vi "Create Reference.vi"(8 "Error In":errorcluster, 11 "Reader In":refnum<class "Reader.lvclass">) -> (0 "Error Out":errorcluster, 3 "Reader Out":refnum<data-value>)   [LabVIEW 2017, in "LabPack.lvlib" / "Reader.lvclass"]
doc: "Creates a Data Value Reference (DVR) of a Reader object. This facilitates a \"pass by reference\"-like approach to using the Reader class. Use this to ensure a single copy of a Reader object exists within an application."
uses:
  Reader.lvclass
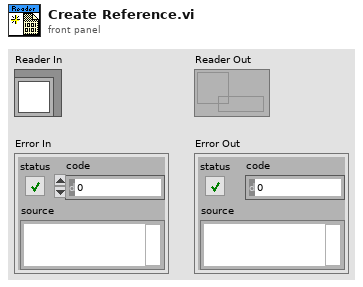
[diagram p1: front panel]
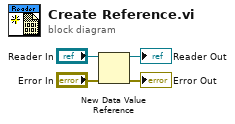
[diagram p0: block diagram]
diagram:
  n1 = New Data Value Reference(data value="Reader In", error in="Error In") -> (data value reference=→"Reader Out":refnum<data-value>, error out=→"Error Out":errorcluster)
